vi "test_F9P_fgv-ver.vi"() -> ()   [LabVIEW 2019] (continued)
09,1*7E\r\n$GLGSV,2,2,06,85,63,111,33,86,51,337,,1*7A\r\n$GLGSV,2,1,06,70,55,030,,71,68,223,25,72,17,216,21,84,09,133,09,3*7F\r\n$GLGSV,2,2,06,85,63,111,25,86,51,337,,3*7F\r\n$GAGSV,3,1,09,02,04,287,06,04,68,085,42,09,44,196,28,11,78,037,38,7*79\r\n$GAGSV,3,2,09,12,32,114,29,18,55,284,36,19,17,042,37,25,01,241,,7*79\r\n$GAGSV,3,3,09,36,34,314,25,7*49\r\n$GAGSV,3,1,09,02,04,287,,04,68,085,36,09,44,196,21,11,78,037,32,2*7A\r\n$GAGSV,3,2,09,12,32,114,24,18,55,284,40,19,17,042,34,25,01,241,,2*73\r\n$GAGSV,3,3,09,36,34,314,19,2*43\r\n$GBGSV,4,1,13,04,35,133,,05,09,257,,06,27,182,,07,09,201,22,1*7B\r\n$GBGSV,4,2,13,08,65,355,40,09,07,194,,10,16,222,17,11,38,142,26,1*76\r\n$GBGSV,4,3,13,13,50,314,21,14,77,038,42,28,58,310,32,33,72,237,31,1*7C\r\n$GBGSV,4,4,13,34,13,141,,1*45\r\n$GBGSV,4,1,13,04,35,133,,05,09,257,,06,27,182,,07,09,201,,3*79\r\n$GBGSV,4,2,13,08,65,355,38,09,07,194,,10,16,222,20,11,38,142,29,3*70\r\n$GBGSV,4,3,13,13,50,314,,14,77,038,40,28,58,310,,33,72,237,,3*7C\r\n$GBGSV,4,4,13,34,13,141,,3*47\r\n$GNGLL,3723.61378,N,12656.96129,E,064232.00,A,A*7B\r\n$GNRMC,064233.00,A,3723.61416,N,12656.96206,E,2.475,72.00,250720,,,A,V*35\r\n$GNVTG,72.00,T,,M,2.475,N,4.584,K,A*1F\r\n$GNGGA,064233.00,3723.61416,N,12656.96206,E,1,12,0.71,43.0,M,18.5,M,,*70\r\n$GNGSA,A,3,17,19,06,05,02,12,09,,,,,,1.15,0.71,0.90,1*0E\r\n$GNGSA,A,3,85,70,71,72,,,,,,,,,1.15,0.71,0.90,2*01\r\n$GNGSA,A,3,36,19,11,04,09,12,,,,,,,1.15,0.71,0.90,3*0A\r\n$GNGSA,A,3,28,14,13,11,33,08,10,,,,,,1.15,0.71,0.90,4*0A\r\n$GPGSV,4,1,13,02,65,334,45,04,08,037,31,05,48,261,36,06,58,076,40,1*6A\r\n$GPGSV,4,2,13,07,06,105,,09,38,057,46,12,18,263,27,13,08,191,21,1*6F\r\n$GPGSV,4,3,13,17,19,158,26,19,37,161,36,25,11,294,18,29,07,323,23,1*66\r\n$GPGSV,4,4,13,30,01,134,,1*52\r\n$GPGSV,4,1,13,02,65,334,,04,08,037,32,05,48,261,37,06,58,076,28,6*60\r\n$GPGSV,4,2,13,07,06,105,,09,38,057,35,12,18,263,16,13,08,191,,6*6D\r\n$GPGSV,4,3,13,17,19,158,20,19,37,161,,25,11,294,,29,07,323,,6*6A\r\n$GPGSV,4,4,13,30,01,134,,6*55\r\n$GLGSV,2,1,06,70,55,030,35,71,68,223,38,72,17,216,25,84,09,133,10,1*7B\r\n$GLGSV,2,2,06,85,63,111,28,86,51,337,,1*70\r\n$GLGSV,2,1,06,70,55,030,,71,68,223,24,72,17,216,21,84,09,133,10,3*76\r\n$GLGSV,2,2,06,85,63,111,26,86,51,337,,3*7C\r\n$GAGSV,3,1,09,02,04,287,09,04,68,085,34,09,44,196,33,11,78,037,37,7*72\r\n$GAGSV,3,2,09,12,32,114,28,18,55,284,30,19,17,042,38,25,01,241,,7*71\r\n$GAGSV,3,3,09,36,34,314,25,7*49\r\n$GAGSV,3,1,09,02,04,287,,04,68,085,31,09,44,196,24,11,78,037,34,2*7E\r\n$GAGSV,3,2,09,12,32,114,25,18,55,284,40,19,17,042,36,25,01,241,,2*70\r\n$GAGSV,3,3,09,36,34,314,21,2*48\r\n$GBGSV,4,1,13,04,35,133,,05,09,257,,06,27,182,,07,09,201,23,1*7A\r\n$GBGSV,4,2,13,08,65,355,39,09,07,194,,10,16,222,17,11,38,142,31,1*7E\r\n$GBGSV,4,3,13,13,50,314,22,14,77,038,38,28,58,310,26,33,72,237,34,1*72\r\n$GBGSV,4,4,13,34,13,141,,1*45\r\n$GBGSV,4,1,13,04,35,133,,05,09,257,,06,27,182,,07,09,201,,3*79\r\n$GBGSV,4,2,13,08,65,355,38,09,07,194,,10,16,222,19,11,38,142,30,3*72\r\n$GBGSV,4,3,13,13,50,314,,14,77,038,38,28,58,310,,33,72,237,,3*73\r\n$GBGSV,4,4,13,34,13,141,,3*47\r\n$GNGLL,3723.61416,N,12656.96206,E,064233.00,A,A*7B\r\n$GNRMC,064234.00,A,3723.61454,N,12656.96282,E,2.658,66.54,250720,,,A,V*31\r\n$GNVTG,66.54,T,,M,2.658,N,4.922,K,A*16\r\n$GNGGA,064234.00,3723.61454,N,12656.96282,E,1,12,0.67,43.2,M,18.5,M,,*78\r\n$GNGSA,A,3,17,19,06,05,02,12,09,,,,,,1.12,0.67,0.90,1*0E\r\n$GNGSA,A,3,85,70,71,72,,,,,,,,,1.12,0.67,0.90,2*01\r\n$GNGSA,A,3,36,19,11,04,09,12,,,,,,,1.12,0.67,0.90,3*0A\r\n$GNGSA,A,3,28,14,13,11,33,08,10,,,,,,1.12,0.67,0.90,4*0A\r\n$GPGSV,4,1,13,02,65,334,45,04,08,037,39,05,48,261,41,06,58,076,40,1*62\r\n$GPGSV,4,2,13,07,06,105,20,09,38,057,41,12,18,263,27,13,08,191,21,1*6A\r\n$GPGSV,4,3,13,17,19,158,31,19,37,161,36,25,11,294,19,29,07,323,21,1*63\r\n$GPGSV,4,4,13,30,01,134,,1*52\r\n$GPGSV,4,1,13,02,65,334,,04,08,037,26,05,48,261,37,06,58,076,33,6*6F\r\n$GPGSV,4,2,13,07,06,105,,09,38,057,37,12,18,263,15,13,08,191,,6*6C\r\n$GPGSV,4,3,13,17,19,158,19,19,37,161,,25,11,294,,29,07,323,,6*60\r\n$GPGSV,4,4,13,30,01,134,,6*55\r\n$GLGSV,2,1,06,70,55,030,25,71,68,223,32,72,17,216,27,84,09,133,12,1*70\r\n$GLGSV,2,2,06,85,63,111,31,86,51,337,,1*78\r\n$GLGSV,2,1,06,70,55,030,,71,68,223,24,72,17,216,21,84,09,133,09,3*7E\r\n$GLGSV,2,2,06,85,63,111,24,86,51,337,,3*7E\r\n$GAGSV,3,1,09,02,04,287,11,04,68,085,30,09,44,196,31,11,78,037,38,7*72\r\n$GAGSV,3,2,09,12,32,114,27,18,55,284,37,19,17,042,32,25,01,241,,7*73\r\n$GAGSV,3,3,09,36,34,314,27,7*4B\r\n$GAGSV,3,1,09,02,04,287,,04,68,085,32,09,44,196,26,11,78,037,30,2*7B\r\n$GAGSV,3,2,09,12,32,114,24,18,55,284,37,19,17,042,37,25,01,241,,2*70\r\n$GAGSV,3,3,09,36,34,314,20,2*49\r\n$GBGSV,4,1,13,04,35,133,,05,09,257,,06,27,182,,07,09,201,29,1*70\r\n$GBGSV,4,2,13,08,65,355,37,09,07,194,,10,16,222,17,11,38,142,29,1*79\r\n$GBGSV,4,3,13,13,50,314,25,14,77,038,36,28,58,310,32,33,72,237,42,1*7F\r\n$GBGSV,4,4,13,34,13,141,,1*45\r\n$GBGSV,4,1,13,04,35,133,,05,09,257,,06,27,182,,07,09,201,,3*79\r\n$GBGSV,4,2,13,08,65,355,35,09,07,194,,10,16,222,19,11,38,142,31,3*7E\r\n$GBGSV,4,3,13,13,50,314,,14,77,038,37,28,58,310,,33,72,237,,3*7C\r\n$GBGSV,4,4,13,34,13,141,,3*47\r\n$GNGLL,3723.61454,N,12656.96282,E,064234.00,A,A*76\r\n$GNRMC,064235.00,A,3723.61480,N,12656.96363,E,2.377,63.39,250720,,,A,V*31\r\n$GNVTG,63.39,T,,M,2.377,N,4.402,K,A*1F\r\n$GNGGA,064235.00,3723.61480,N,12656.96363,E,1,12,0.63,43.0,M,18.5,M,,*78\r\n$GNGSA,A,3,17,19,06,05,02,12,09,,,,,,1.08,0.63,0.88,1*08\r\n$GNGSA,A,3,85,70,71,72,,,,,,,,,1.08,0.63,0.88,2*07\r\n$GNGSA,A,3,36,19,11,04,09,12,,,,,,,1.08,0.63,0.88,3*0C\r\n$GNGSA,A,3,28,14,13,11,33,08,10,,,,,,1.08,0.63,0.88,4*0C\r\n$GPGSV,4,1,13,02,65,334,42,04,08,037,41,05,48,261,38,06,58,076,39,1*6A\r\n$GPGSV,4,2,13,07,06,105,19,09,38,057,36,12,18,263,32,13,08,191,20,1*65\r\n$GPGSV,4,3,13,17,19,158,31,19,37,161,36,25,11,294,20,29,07,323,20,1*68\r\n$GPGSV,4,4,13,30,01,134,,1*52\r\n$GPGSV,4,1,13,02,65,334,,04,08,037,31,05,48,261,37,06,58,076,33,6*69\r\n$GPGSV,4,2,13,07,06,105,,09,38,057,38,12,18,263,14,13,08,191,,6*62\r\n$GPGSV,4,3,13,17,19,158,20,19,37,161,,25,11,294,,29,07,323,,6*6A\r\n$GPGSV,4,4,13,30,01,134,,6*55\r\n$GLGSV,2,1,06,70,55,030,32,71,68,223,31,72,17,216,32,84,09,133,11,1*72\r\n$GLGSV,2,2,06,85,63,111,30,86,51,337,,1*79\r\n$GLGSV,2,1,06,70,55,030,,71,68,223,24,72,17,216,23,84,09,133,09,3*7C\r\n$GLGSV,2,2,06,85,63,111,23,86,51,337,,3*79\r\n$GAGSV,3,1,09,02,04,287,09,04,68,085,33,09,44,196,31,11,78,037,34,7*74\r\n$GAGSV,3,2,09,12,32,114,27,18,55,284,32,19,17,042,30,25,01,241,,7*74\r\n$GAGSV,3,3,09,36,34,314,31,7*4C\r\n$GAGSV,3,1,09,02,04,287,,04,68,085,34,09,44,196,32,11,78,037,30,2*78\r\n$GAGSV,3,2,09,12,32,114,25,18,55,284,39,19,17,042,34,25,01,241,,2*7C\r\n$GAGSV,3,3,09,36,34,314,18,2*42\r\n$GBGSV,4,1,13,04,35,133,,05,09,257,,06,27,182,,07,09,201,25,1*7C\r\n$GBGSV,4,2,13,08,65,355,39,09,07,194,,10,16,222,17,11,38,142,21,1*7F\r\n$GBGSV,4,3,13,13,50,314,26,14,77,038,37,28,58,310,32,33,72,237,31,1*79\r\n$GBGSV,4,4,13,34,13,141,,1*45\r\n$GBGSV,4,1,13,04,35,133,,05,09,257,,06,27,182,,07,09,201,,3*79\r\n$GBGSV,4,2,13,08,65,355,38,09,07,194,,10,16,222,20,11,38,142,26,3*7F\r\n$GBGSV,4,3,13,13,50,314,31,14,77,038,34,28,58,310,,33,72,237,,3*7D\r\n$GBGSV,4,4,13,34,13,141,,3*47\r\n$GNGLL,3723.61480,N,12656.96363,E,064235.00,A,A*70\r\n$GNRMC,064236.00,A,3723.61511,N,12656.96445,E,2.628,61.27,250720,,,A,V*3A\r\n$GNVTG,61.27,T,,M,2.628,N,4.867,K,A*12\r\n$GNGGA,064236.00,3723.61511,N,12656.96445,E,1,12,0.65,42.8,M,18.5,M,,*7E\r\n$GNGSA,A,3,17,19,06,05,02,12,09,,,,,,1.12,0.65,0.91,1*0D\r\n$GNGSA,A,3,85,70,71,72,,,,,,,,,1.12,0.65,0.91,2*02\r\n$GNGSA,A,3,36,19,11,04,09,12,,,,,,,1.12,0.65,0.91,3*09\r\n$GNGSA,A,3,28,14,13,11,33,08,10,,,,,,1.12,0.65,0.91,4*09\r\n$GPGSV,4,1,13,02,65,334,41,04,08,037,35,05,48,261,38,06,58,076,40,1*64\r\n$GPGSV,4,2,13,07,06,105,,09,38,057,40,12,18,263,25,13,08,191,,1*68\r\n$GPGSV,4,3,13,17,19,158,25,19,37,161,34,25,11,294,19,29,07,323,19,1*6F\r\n$GPGSV,4,4,13,30,01,134,,1*52\r\n$GPGSV,4,1,13,02,65,334,,04,08,037,31,05,48,261,35,06,58,076,27,6*6E\r\n$GPGSV,4,2,13,07,06,105,,09,38,057,39,12,18,263,12,13,08,191,,6*65\r\n$GPGSV,4,3,13,17,19,158,21,19,37,161,,25,11,294,,29,07,323,,6*6B\r\n$GPGSV,4,4,13,30,01,134,,6*55\r\n$GLGSV,2,1,06,70,55,030,27,71,68,223,33,72,17,216,36,84,09,133,08,1*78\r\n$GLGSV,2,2,06,85,63,111,37,86,51,337,,1*7E\r\n$GLGSV,2,1,06,70,55,030,,71,68,223,23,72,17,216,31,84,09,133,10,3*70\r\n$GLGSV,2,2,06,85,63,111,24,86,51,337,,3*7E\r\n$GAGSV,3,1,09,02,04,287,09,04,68,085,36,09,44,196,24,11,78,037,34,7*75\r\n$GAGSV,3,2,09,12,32,114,32,18,55,284,36,19,17,042,40,25,01,241,,7*73\r\n$GAGSV,3,3,09,36,35,314,27,7*4A\r\n$GAGSV,3,1,09,02,04,287,,04,68,085,31,09,44,196,31,11,78,037,29,2*76\r\n$GAGSV,3,2,09,12,32,114,25,18,55,284,35,19,17,042,31,25,01,241,,2*75\r\n$GAGSV,3,3,09,36,35,314,19,2*42\r\n$GBGSV,4,1,13,04,35,133,,05,09,257,,06,27,182,,07,09,201,24,1*7D\r\n$GBGSV,4,2,13,08,65,355,38,09,07,194,,10,16,222,17,11,38,142,,1*7D\r\n$GBGSV,4,3,13,13,50,314,34,14,77,038,35,28,58,310,36,33,72,237,35,1*78\r\n$GBGSV,4,4,13,34,13,141,,1*45\r\n$GBGSV,4,1,13,04,35,133,,05,09,257,,06,27,182,,07,09,201,,3*79\r\n$GBGSV,4,2,13,08,65,355,38,09,07,194,,10,16,222,18,11,38,142,28,3*7A\r\n$GBGSV,4,3,13,13,50,314,27,14,77,038,33,28,58,310,,33,72,237,,3*7D\r\n$GBGSV,4,4,13,34,13,141,,3*47\r\n$GNGLL,3723.61511,N,12656.96445,E,064236.00,A,A*79\r\n$GNRMC,064237.00,A,3723.61540,N,12656.96523,E,2.163,60.56,250720,,,A,V*31\r\n$GNVTG,60.56,T,,M,2.163,N,4.005,K,A*11\r\n$GNGGA,064237.00,3723.61540,N,12656.96523,E,1,12,0.63,42.6,M,18.5,M,,*72\r\n$GNGSA,A,3,17,19,06,05,02,12,09,,,,,,1.11,0.63,0.91,1*08\r\n$GNGSA,A,3,85,70,71,72,,,,,,,,,1.11,0.63,0.91,2*07\r\n$GNGSA,A,3,36,19,11,04,09,12,,,,,,,1.11,0.63,0.91,3*0C\r\n$GNGSA,A,3,28,14,13,11,33,08,10,,,,,,1.11,0.63,0.91,4*0C\r\n$GPGSV,4,1,13,02,65,334,41,04,08,037,40,05,48,261,37,06,58,076,44,1*6D\r\n$GPGSV,4,2,13,07,06,105,,09,38,057,45,12,18,263,24,13,08,191,21,1*6F\r\n$GPGSV,4,3,13,17,19,158,26,19,37,161,28,25,11,294,19,29,07,323,18,1*60\r\n$GPGSV,4,4,13,30,01,134,,1*52\r\n$GPGSV,4,1,13,02,65,334,,04,08,037,34,05,48,261,29,06,58,076,35,6*65\r\n$GPGSV,4,2,13,07,06,105,,09,38,057,39,12,18,263,13,13,08,191,,6*64\r\n$GPGSV,4,3,13,17,19,158,20,19,37,161,,25,11,294,,29,07,323,,6*6A\r\n$GPGSV,4,4,13,30,01,134,,6*55\r\n$GLGSV,2,1,06,70,55,030,31,71,68,223,31,72,17,216,36,84,09,133,12,1*76\r\n$GLGSV,2,2,06,85,63,111,31,86,51,337,,1*78\r\n$GLGSV,2,1,06,70,55,030,,71,68,223,24,72,17,216,30,84,09,133,11,3*77\r\n$GLGSV,2,2,06,85,63,111,26,86,51,337,,3*7C\r\n$GAGSV,3,1,09,02,04,287,07,04,68,085,33,09,44,196,30,11,78,037,31,7*7E\r\n$GAGSV,3,2,09,12,32,114,31,18,55,284,36,19,17,042,35,25,01,241,,7*72\r\n$GAGSV,3,3,09,36,35,314,36,7*4A\r\n$GAGSV,3,1,09,02,04,287,,04,68,085,35,09,44,196,25,11,78,037,29,2*77\r\n$GAGSV,3,2,09,12,32,114,25,18,55,284,38,19,17,042,30,25,01,241,,2*79\r\n$GAGSV,3,3,09,36,35,314,36,2*4F\r\n$GBGSV,4,1,13,04,35,133,,05,09,257,,06,27,182,,07,09,201,24,1*7D\r\n$GBGSV,4,2,13,08,65,355,36,09,07,194,,10,16,222,19,11,38,142,30,1*7E\r\n$GBGSV,4,3,13,13,50,314,39,14,77,038,35,28,58,310,37,33,72,237,34,1*75\r\n$GBGSV,4,4,13,34,13,141,,1*45\r\n$GBGSV,4,1,13,04,35,133,,05,09,257,,06,27,182,,07,09,201,,3*79\r\n$GBGSV,4,2,13,08,65,355,37,09,07,194,,10,16,222,20,11,38,142,33,3*74\r\n$GBGSV,4,3,13,13,50,314,32,14,77,038,37,28,58,310,,33,72,237,,3*7D\r\n$GBGSV,4,4,13,34,13,141,,3*47\r\n$GNGLL,3723.61540,N,12656.96523,E,064237.00,A,A*7D\r\n$GNRMC,064238.00,A,3723.61556,N,12656.96586,E,1.985,69.85,250720,,,A,V*32\r\n$GNVTG,69.85,T,,M,1.985,N,3.676,K,A*10\r\n$GNGGA,064238.00,3723.61556,N,12656.96586,E,1,12,0.62,41.9,M,18.5,M,,*78\r\n$GNGSA,A,3,17,19,06,05,02,12,09,,,,,,1.07,0.62,0.88,1*06\r\n$GNGSA,A,3,85,70,71,72,,,,,,,,,1.07,0.62,0.88,2*09\r\n$GNGSA,A,3,36,19,11,04,09,12,,,,,,,1.07,0.62,0.88,3*02\r\n$GNGSA,A,3,28,14,13,11,33,08,10,,,,,,1.07,0.62,0.88,4*02\r\n$GPGSV,4,1,13,02,65,334,38,04,08,037,43,05,48,261,32,06,58,076,42,1*63\r\n$GPGSV,4,2,13,07,06,105,,09,38,057,42,12,18,263,24,13,08,191,,1*6B\r\n$GPGSV,4,3,13,17,19,158,26,19,37,161,28,25,11,294,18,29,07,323,17,1*6E\r\n$GPGSV,4,4,13,30,01,134,,1*52\r\n$GPGSV,4,1,13,02,65,334,,04,08,037,33,05,48,261,33,06,58,076,32,6*6E\r\n$GPGSV,4,2,13,07,06,105,,09,38,057,34,12,18,263,14,13,08,191,,6*6E\r\n$GPGSV,4,3,13,17,19,158,19,19,37,161,,25,11,294,,29,07,323,,6*60\r\n$GPGSV,4,4,13,30,01,134,,6*55\r\n$GLGSV,2,1,06,70,55,030,31,71,68,223,31,72,17,216,39,84,09,133,12,1*79\r\n$GLGSV,2,2,06,85,63,111,37,86,51,337,,1*7E\r\n$GLGSV,2,1,06,70,55,030,,71,68,223,23,72,17,216,30,84,09,133,10,3*71\r\n$GLGSV,2,2,06,85,63,111,26,86,51,337,,3*7C\r\n$GAGSV,3,1,09,02,04,287,12,04,68,085,32,09,44,196,23,11,78,037,33,7*7B\r\n$GAGSV,3,2,09,12,32,114,34,18,55,284,33,19,17,042,40,25,01,241,,7*70\r\n$GAGSV,3,3,09,36,35,314,35,7*49\r\n$GAGSV,3,1,09,02,04,287,,04,68,085,35,09,44,196,25,11,78,037,30,2*7F\r\n$GAGSV,3,2,09,12,32,114,31,18,55,284,30,19,17,042,25,25,01,241,,2*70\r\n$GAGSV,3,3,09,36,35,314,35,2*4C\r\n$GBGSV,4,1,13,04,35,133,,05,09,257,,06,27,182,,07,09,201,23,1*7A\r\n$GBGSV,4,2,13,08,65,355,37,09,07,194,,10,16,222,20,11,38,142,31,1*74\r\n$GBGSV,4,3,13,13,50,314,38,14,77,038,38,28,58,310,42,33,72,237,34,1*7B\r\n$GBGSV,4,4,13,34,13,141,,1*45\r\n$GBGSV,4,1,13,04,35,133,,05,09,257,,06,27,182,,07,09,201,,3*79\r\n$GBGSV,4,2,13,08,65,355,34,09,07,194,,10,16,222,19,11,38,142,26,3*79\r\n$GBGSV,4,3,13,13,50,314,34,14,77,038,36,28,58,310,,33,72,237,,3*7A\r\n$GBGSV,4,4,13,34,13,141,,3*47\r\n$GNGLL,3723.61556,N,12656.96586,E,064238.00,A,A*7A\r\n$GNRMC,064239.00,A,3723.61573,N,12656.96659,E,1.968,70.42,250720,,,A,V*35\r\n$GNVTG,70.42,T,,M,1.968,N,3.646,K,A*13\r\n$GNGGA,064239.00,3723.61573,N,12656.96659,E,1,12,0.65,41.7,M,18.5,M,,*76\r\n$GNGSA,A,3,17,19,06,05,02,12,09,,,,,,1.18,0.65,0.98,1*0E\r\n$GNGSA,A,3,85,70,71,72,,,,,,,,,1.18,0.65,0.98,2*01\r\n$GNGSA,A,3,36,19,11,04,09,12,,,,,,,1.18,0.65,0.98,3*0A\r\n$GNGSA,A,3,28,14,13,11,33,08,10,,,,,,1.18,0.65,0.98,4*0A\r\n$GPGSV,4,1,13,02,65,334,42,04,08,037,42,05,48,261,44,06,58,076,44,1*68\r\n$GPGSV,4,2,13,07,06,105,,09,38,057,45,12,18,263,23,13,08,191,,1*6B\r\n$GPGSV,4,3,13,17,19,158,26,19,37,161,27,25,11,294,18,29,07,323,18,1*6E\r\n$GPGSV,4,4,13,30,01,134,,1*52\r\n$GPGSV,4,1,13,02,65,334,,04,08,037,29,05,48,261,31,06,58,076,38,6*6D\r\n$GPGSV,4,2,13,07,06,105,,09,38,057,40,12,18,263,15,13,08,191,,6*6C\r\n$GPGSV,4,3,13,17,19,158,20,19,37,161,,25,11,294,,29,07,323,,6*6A\r\n$GPGSV,4,4,13,30,01,134,,6*55\r\n$GLGSV,2,1,06,70,55,030,35,71,68,223,37,72,17,216,37,84,09,133,11,1*76\r\n$GLGSV,2,2,06,85,63,111,31,86,51,337,,1*78\r\n$GLGSV,2,1,06,70,55,030,,71,68,223,23,72,17,216,30,84,09,133,12,3*73\r\n$GLGSV,2,2,06,85,63,111,24,86,51,337,,3*7E\r\n$GAGSV,3,1,09,02,04,287,13,04,68,085,40,09,44,196,33,11,78,037,34,7*79\r\n$GAGSV,3,2,09,12,32,114,30,18,55,284,29,19,17,042,38,25,01,241,,7*70\r\n$GAGSV,3,3,09,36,35,314,29,7*44\r\n$GAGSV,3,1,09,02,04,287,,04,68,085,30,09,44,196,25,11,78,037,31,2*7B\r\n$GAGSV,3,2,09,12,32,114,24,18,55,284,34,19,17,042,34,25,01,241,,2*70\r\n$GAGSV,3,3,09,36,35,314,25,2*4D\r\n$GBGSV,4,1,13,04,35,133,,05,09,257,,06,27,182,,07,09,201,26,1*7F\r\n$GBGSV,4,2,13,08,65,355,39,09,07,194,,10,16,222,20,11,38,142,27,1*7D\r\n$GBGSV,4,3,13,13,50,314,32,14,77,038,38,28,58,310,39,33,72,237,36,1*7F\r\n$GBGSV,4,4,13,34,13,141,,1*45\r\n$GBGSV,4,1,13,04,35,133,,05,09,257,,06,27,182,,07,09,201,,3*79\r\n$GBGSV,4,2,13,08,65,355,36,09,07,194,,10,16,222,18,11,38,142,31,3*7C\r\n$GBGSV,4,3,13,13,50,314,31,14,77,038,36,28,58,310,,33,72,237,,3*7F\r\n$GBGSV,4,4,13,34,13,141,,3*47\r\n$GNGLL,3723.61573,N,12656.96659,E,064239.00,A,A*7D\r\n$GNRMC,064240.00,A,3723.61583,N,12656.96722,E,1.594,75.78,250720,,,A,V*3A\r\n$GNVTG,75.78,T,,M,1.594,N,2.952,K,A*1B\r\n$GNGGA,064240.00,3723.61583,N,12656.96722,E,1,12,0.64,41.6,M,18.5,M,,*7A\r\n$GNGSA,A,3,17,19,06,05,02,12,09,,,,,,1.13,0.64,0.93,1*0F\r\n$GNGSA,A,3,85,70,71,72,,,,,,,,,1.13,0.64,0.93,2*00\r\n$GNGSA,A,3,36,19,11,04,09,12,,,,,,,1.13,0.64,0.93,3*0B\r\n$GNGSA,A,3,28,14,13,11,33,08,10,,,,,,1.13,0.64,0.93,4*0B\r\n$GPGSV,4,1,13,02,65,334,41,04,08,037,42,05,48,261,39,06,58,076,45,1*60\r\n$GPGSV,4,2,13,07,06,105,,09,38,057,46,12,18,263,22,13,08,191,,1*69\r\n$GPGSV,4,3,13,17,19,158,35,19,37,161,32,25,11,294,17,29,07,323,19,1*66\r\n$GPGSV,4,4,13,30,01,134,,1*52\r\n$GPGSV,4,1,13,02,65,334,,04,08,037,21,05,48,261,25,06,58,076,30,6*68\r\n$GPGSV,4,2,13,07,06,105,,09,38,057,37,12,18,263,15,13,08,191,,6*6C\r\n$GPGSV,4,3,13,17,19,158,19,19,37,161,,25,11,294,,29,07,323,,6*60\r\n$GPGSV,4,4,13,30,01,134,,6*55\r\n$GLGSV,2,1,06,70,55,030,34,71,68,223,30,72,17,216,35,84,09,133,14,1*77\r\n$GLGSV,2,2,06,85,63,111,34,86,51,337,,1*7D\r\n$GLGSV,2,1,06,70,55,030,,71,68,223,23,72,17,216,24,84,09,133,11,3*75\r\n$GLGSV,2,2,06,85,63,111,24,86,51,337,,3*7E\r\n$GAGSV,3,1,09,02,04,287,08,04,68,085,39,09,44,196,29,11,78,037,37,7*75\r\n$GAGSV,3,2,09,12,32,114,24,18,55,284,33,19,17,042,38,25,01,241,,7*7E\r\n$GAGSV,3,3,09,36,35,314,21,7*4C\r\n$GAGSV,3,1,09,02,04,287,,04,68,085,31,09,44,196,26,11,78,037,29,2*70\r\n$GAGSV,3,2,09,12,32,114,35,18,55,284,26,19,17,042,31,25,01,241,,2*76\r\n$GAGSV,3,3,09,36,35,314,25,2*4D\r\n$GBGSV,4,1,13,04,35,133,,05,09,257,,06,27,182,,07,09,201,24,1*7D\r\n$GBGSV,4,2,13,08,65,355,38,09,07,194,,10,16,222,19,11,38,142,27,1*76\r\n$GBGSV,4,3,13,13,50,314,38,14,77,038,41,28,58,310,35,33,72,237,29,1*79\r\n$GBGSV,4,4,13,34,13,141,,1*45\r\n$GBGSV,4,1,13,04,35,133,,05,09,257,,06,27,182,,07,09,201,,3*79\r\n$GBGSV,4,2,13,08,65,355,35,09,07,194,,10,16,222,17,11,38,142,25,3*75\r\n$GBGSV,4,3,13,13,50,314,34,14,77,038,36,28,58,310,,33,72,237,,3*7A\r\n$GBGSV,4,4,13,34,13,141,,3*47\r\n$GNGLL,3723.61583,N,12656.96722,E,064240.00,A,A*71\r\n$GNRMC,064241.00,A,3723.61598,N,12656.96755,E,0.627,70.48,250720,,,A,V*3D\r\n$GNVTG,70.48,T,,M,0.627,N,1.162,K,A*1F\r\n$GNGGA,064241.00,3723.61598,N,12656.96755,E,1,12,0.67,41.6,M,18.5,M,,*72\r\n$GNGSA,A,3,17,19,06,05,02,12,09,,,,,,1.19,0.67,0.98,1*0D\r\n$GNGSA,A,3,85,70,71,72,,,,,,,,,1.19,0.67,0.98,2*02\r\n$GNGSA,A,3,36,19,11,04,09,12,,,,,,,1.19,0.67,0.98,3*09\r\n$GNGSA,A,3,28,14,13,11,33,08,10,,,,,,1.19,0.67,0.98,4*09\r\n$GPGSV,4,1,13,02,65,334,43,04,08,037,43,05,48,261,37,06,58,076,41,1*69\r\n$GPGSV,4,2,13,07,06,105,28,09,38,057,43,12,18,263,22,13,08,191,,1*66\r\n$GPGSV,4,3,13,17,19,158,26,19,37,161,34,25,11,294,17,29,07,323,20,1*68\r\n$GPGSV,4,4,13,30,01,134,,1*52\r\n$GPGSV,4,1,13,02,65,334,,04,08,037,20,05,48,261,32,06,58,076,23,6*6D\r\n$GPGSV,4,2,13,07,06,105,,09,38,057,35,12,18,263,14,13,08,191,,6*6F\r\n$GPGSV,4,3,13,17,19,158,18,19,37,161,,25,11,294,,29,07,323,,6*61\r\n$GPGSV,4,4,13,30,01,134,,6*55\r\n$GLGSV,2,1,06,70,55,030,37,71,68,223,33,72,17,216,39,84,09,133,13,1*7C\r\n$GLGSV,2,2,06,85,63,111,34,86,51,337,,1*7D\r\n$GLGSV,2,1,06,70,55,030,,71,68,223,20,72,17,216,24,84,09,133,08,3*7E\r\n$GLGSV,2,2,06,85,63,111,24,86,51,337,,3*7E\r\n$GAGSV,3,1,09,02,04,287,09,04,68,085,40,09,44,196,28,11,78,037,37,7*7B\r\n$GAGSV,3,2,09,12,32,114,25,18,55,284,38,19,17,042,38,25,01,241,,7*74\r\n$GAGSV,3,3,09,36,35,314,30,7*4C\r\n$GAGSV,3,1,09,02,04,287,,04,68,085,33,09,44,196,26,11,78,037,30,2*7A\r\n$GAGSV,3,2,09,12,32,114,28,18,55,284,33,19,17,042,32,25,01,241,,2*7D\r\n$GAGSV,3,3,09,36,35,314,25,2*4D\r\n$GBGSV,4,1,13,04,35,133,,05,09,257,,06,27,182,,07,09,201,23,1*7A\r\n$GBGSV,4,2,13,08,65,355,40,09,07,194,,10,16,222,19,11,38,142,32,1*7D\r\n$GBGSV,4,3,13,13,50,314,41,14,77,038,40,28,58,310,41,33,72,237,30,1*7D\r\n$GBGSV,4,4,13,34,13,141,,1*45\r\n$GBGSV,4,1,13,04,35,133,,05,09,257,,06,27,182,,07,09,201,,3*79\r\n$GBGSV,4,2,13,08,65,355,36,09,07,194,,10,16,222,18,11,38,142,32,3*7F\r\n$GBGSV,4,3,13,13,50,314,39,14,77,038,38,28,58,310,,33,72,237,,3*79\r\n$GBGSV,4,4,13,34,13,141,,3*47\r\n$GNGLL,3723.61598,N,12656.96755,E,064241.00,A,A*7A\r\n$GNRMC,064242.00,A,3723.61598,N,12656.96764,E,0.205,,250720,,,A,V*1D\r\n$GNVTG,,T,,M,0.205,N,0.379,K,A*37\r\n$GNGGA,064242.00,3723.61598,N,12656.96764,E,1,12,0.67,41.4,M,18.5,M,,*71\r\n$GNGSA,A,3,17,19,06,05,02,12,09,,,,,,1.19,0.67,0.98,1*0D\r\n$GNGSA,A,3,85,70,71,72,,,,,,,,,1.19,0.67,0.98,2*02\r\n$GNGSA,A,3,36,19,11,04,09,12,,,,,,,1.19,0.67,0.98,3*09\r\n$GNGSA,A,
